vi "Trim Signals.vi"(8 "error in (no error)":errorcluster, 11 "Signal In":refnum<k21>[](array[refnum])) -> (0 "error out (no error) 2":errorcluster, 3 "Signal Out":refnum<k21>[](array[refnum]))   [LabVIEW 2024]
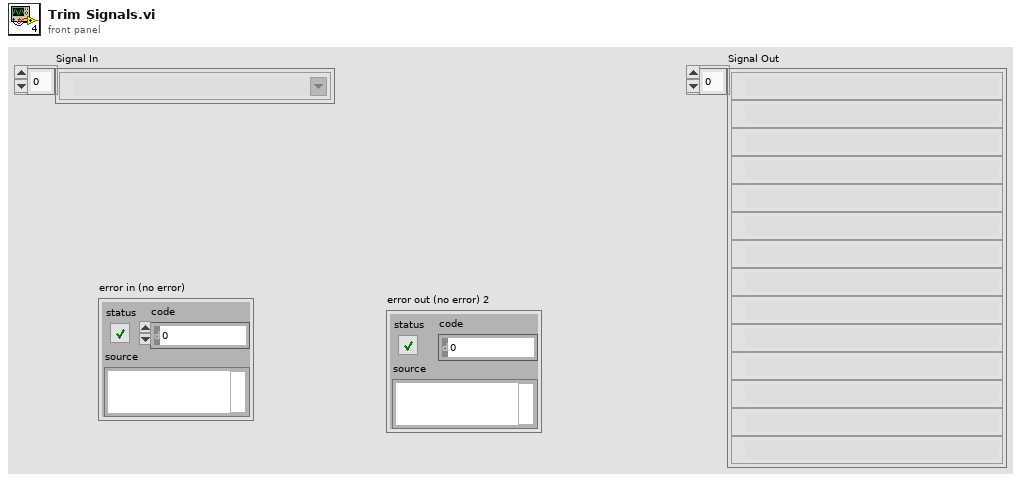
[diagram p1: front panel]
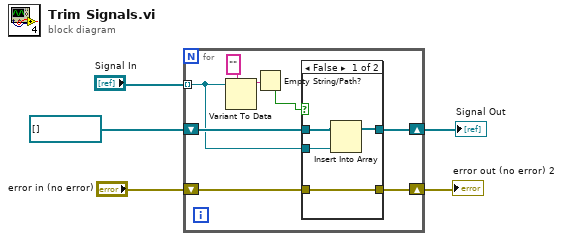
[diagram p0: block diagram]
diagram:
  n1 = for {
    tunnel: "Signal In" -> [w8] mode=indexing
    shift-right: [w9] -> w4
    shift-left: refnum<k21>[] [] -> [w10]
    shift-right: [w6] -> w1
    shift-left: "error in (no error)" -> [w7]
    n2 = Variant To Data(type="", Variant=w8) -> (data=w12:string)  [unwired: 1 in, 1 out]
    n3 = Empty String/Path?(string/path=w12) -> (empty?=w11:bool)
    n4 = case shown="False" w11 {
      tunnel: w10 -> [w17 w19]
      tunnel: [w15 w19] -> w9
      tunnel: w8 -> [w16 _]
      tunnel: w7 -> [w14 w18]
      tunnel: [w14 w18] -> w6
      frame False {
        n5 = Insert Into Array(array=w17, new element=w16) -> (w15:refnum<k21>[])  [unwired: 1 in]
      }
      frame True {
      }
    }
  }
  "Signal Out" <- w4
  "error out (no error) 2" <- w1
